vi "random.vi"(1 "Input":i32[](array[numeric])=[0, 1, 2, 3, 4, 5, 6, 7, 8, 9]) -> (0 "output":i32[](array[numeric]))   [LabVIEW 2014]
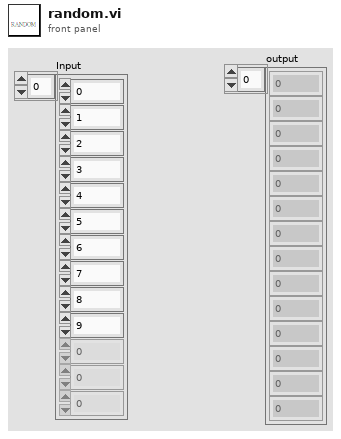
[diagram p1: front panel]
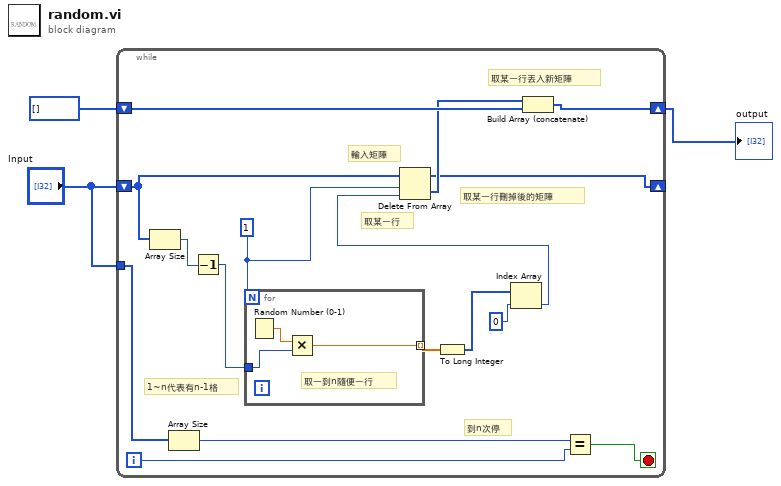
[diagram p0: block diagram]
diagram:
  n1 = while {
    shift-right: [w9] -> w1
    shift-left: i32[] [] -> [w10]
    shift-right: [w4] -> _
    shift-left: "Input" -> [w7]
    tunnel: "Input" -> [w17]
    i -> [w18]
    stop <- w19 stop-if-true
    w6 = 1
    # "取某一行刪掉後的矩陣"
    # "取某一行丟入新矩陣"
    # "取某一行"
    # "輸入矩陣"
    # "1~n代表有n-1格"
    # "到n次停"
    n2 = Array Size(array=w7) -> (size(s)=w15:i32)
    n3 = Array Size(array=w17) -> (size(s)=w16:i32)
    n4 = Decrement(x=w15) -> (x-1=w14:i32)
    n5 = for {
      N: w6 -> [_]
      tunnel: w14 -> [w22]
      tunnel: [w20] -> w13 mode=indexing
      # "取一到n隨便一行"
      n6 = Random Number (0-1)() -> (number: 0 to 1=w21:dbl)
      n7 = Multiply(x=w21, y=w22) -> (x*y=w20:dbl)
    }
    n8 = To Long Integer(number=w13) -> (32bit integer=w12:i32[])
    n9 = Index Array(array=w12, index=0) -> (element=w8:i32)
    n10 = Delete From Array(array=w7, length=w6, index=w8) -> (deleted portion=w5:i32[], array with subset deleted=w4:i32[])
    n11 = Build Array (concatenate)(w5, w10) -> (w9:i32[])
    n12 = Equal?(x=w16, y=w18) -> (x = y?=w19:bool)
  }
  "output" <- w1
